vi "PC_Pub_imgFile markTableRow.vi"(0 "Row":i32, 1 "tableRefNum":refnum<vi>) -> ()   [LabVIEW 2018, in "PC_Pub_imgFile.lvclass"]
uses:
  PC_Pub_imgFile.lvclass
  <vilib>/Utility/miscctls.llb/LVRowAndColumnTypeDef.ctl
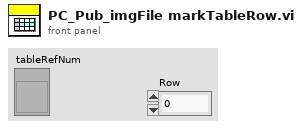
[diagram p1: front panel]
types:
  T1 = typedef "LVRowAndColumnTypeDef.ctl" = cluster{"Row":i32, "Column":i32}
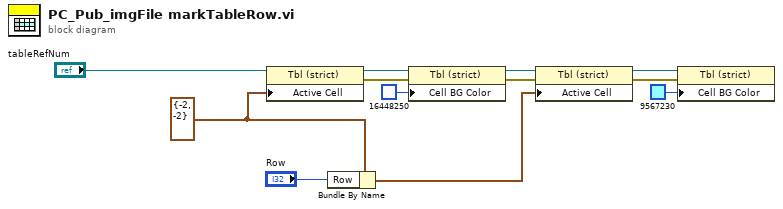
[diagram p0: block diagram]
diagram:
  w12 = T1 {"Row"=-2, "Column"=-2} ("Active Cell:Active Cell")
  n1 = property class="Tbl (strict)"(reference="tableRefNum", "Active Cell"=w12) -> (reference out=w11:refnum<vi>, error out=w10:errorcluster)  [unwired: 1 in]
  n2 = Bundle By Name(cluster=w12, "Row"="Row") -> (w3:T1)
  n3 = property class="Tbl (strict)"(reference=w11, error in=w10, "Cell BG Color"=u32 16448250) -> (reference out=w5:refnum<vi>, error out=w4:errorcluster)
  n4 = property class="Tbl (strict)"(reference=w5, error in=w4, "Active Cell"=w3) -> (reference out=w8:refnum<vi>, error out=w7:errorcluster)
  n5 = property class="Tbl (strict)"(reference=w8, error in=w7, "Cell BG Color"=u32 9567230) -> ()  [unwired: 2 out]
